vi "LOGO V3-Labview-modbus-TCP.vi"() -> ()   [LabVIEW 2023]
uses:
  <vilib>/NI/Modbus Library/API/Wrapper/Create TCP Master.vi
  <vilib>/NI/Modbus Library/API/Master/Modbus Master.lvclass
  <vilib>/NI/Modbus Library/API/Wrapper/API Main.lvlib
panel:
  in  "coil to write":bool
  out "AI1":u16
  out "Q2":bool
  out "Q1":bool
  out "I2":bool
  out "I1":bool
  in  "Write Single Coil":u16
  in  "Port (502)":u16=502
  in  "Ip Address":string="192.168.0.3"
  in  "stop":bool
  # "Loop status"
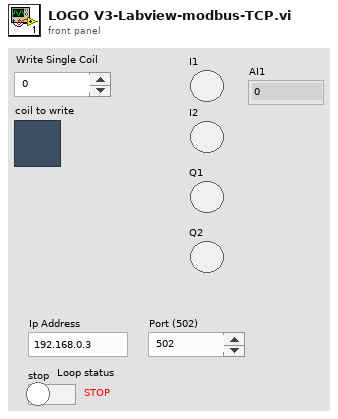
[diagram p1: front panel]
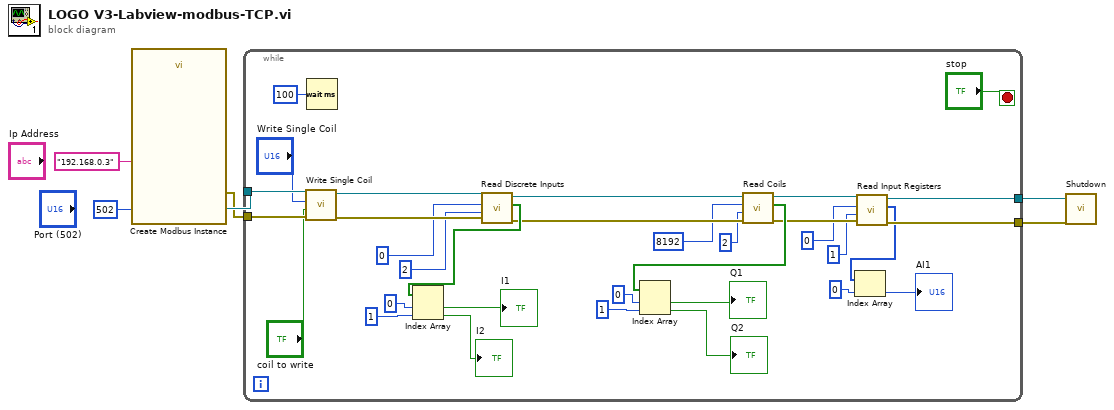
[diagram p0: block diagram]
diagram:
  n1 = call-poly <vilib>:"Create Modbus Instance.vi"("port (502)"=u16 502, "address"="192.168.0.3") -> ("error out"=w3:errorcluster, "TCP master instance"=w4:refnum<class "Modbus Master.lvclass">)  [unwired: 8 in]
  n2 = while {
    tunnel: w4 -> [w37]
    tunnel: w3 -> [w36]
    tunnel: [w12] -> w2
    tunnel: [w11] -> w1
    stop <- "stop" stop-if-true
    n3 = call-dynamic "Write Single Coil.vi"("error in"=w36, "coil to write"="coil to write", "address"="Write Single Coil", "Modbus master in"=w37) -> ("error out"=w33:errorcluster, "Modbus master out"=w34:refnum<class "Modbus Master.lvclass">)  [unwired: 6 in]
    n4 = Wait (ms)(milliseconds to wait=u32 100) -> ()  [unwired: 1 out]
    n5 = call-dynamic "Read Discrete Inputs.vi"("error in"=w33, "number of inputs"=u16 2, "starting address"=u16 0, "Modbus master in"=w34) -> ("error out"=w24:errorcluster, "discrete inputs"=w30:bool[], "Modbus master out"=w25:refnum<class "Modbus Master.lvclass">)  [unwired: 5 in]
    n6 = Index Array(array=w30, index #1=0 ("index"), index #2=1 ("index")) -> (element #1=→"I1":bool, element #2=→"I2":bool)
    n7 = call-dynamic "Read Coils.vi"("error in"=w24, "number of inputs"=u16 2, "starting address"=u16 8192, "Modbus master in"=w25) -> ("error out"=w15:errorcluster, "coils"=w19:bool[], "Modbus master out"=w16:refnum<class "Modbus Master.lvclass">)  [unwired: 5 in]
    n8 = Index Array(array=w19, index #1=0 ("index"), index #2=1 ("index")) -> (element #1=→"Q1":bool, element #2=→"Q2":bool)
    n9 = call-dynamic "Read Input Registers.vi"("error in"=w15, "number of inputs"=u16 1, "starting address"=u16 0, "Modbus master in"=w16) -> ("error out"=w11:errorcluster, "register values"=w9:u16[], "Modbus master out"=w12:refnum<class "Modbus Master.lvclass">)  [unwired: 5 in]
    n10 = Index Array(array=w9, index=0) -> (element=→"AI1":u16)
  }
  n11 = call-dynamic "Shutdown.vi"("error in"=w1, "Modbus master in"=w2) -> ()  [unwired: 9 in, 1 out]
